vi "svfa_Process FRF (N pairs).vi"(0 "stimulus signals X [EUx]":waveform(dbl)[](array[waveform]), 1 "response signals Y [EUy]":waveform(dbl)[](array[waveform]), 2 "window":T9=1 items=["None"=0, "Hanning"=1, "Hamming"=2, "Blackman-Harris"=3, "Exact Blackman"=4, "Blackman"=5, "Flat Top"=6, "4 Term B-Harris "=7, "7 Term B-Harris"=8, "Low Sidelobe"=9, "Force - Exponential"=10, "Blackman Nuttall"=11, "Triangle"=30, "Bartlett-Hanning"=31, "Bohman"=32, "Parzen"=33, "Welch"=34, "Kaiser"=60, "Dolph-Chebyshev"=61, "Gaussian"=62], 3 "force/exp settings":T8={"force window [%]"=50.0, "exp window [%]"=10.0} {"exp window [%]" min=0.0 max=100.0 format="%.2f"; "force window [%]" min=0.0 max=100.0 format="%.2f"}, 4 "averaging parameters":T11={"averaging mode"=enum."No averaging", "weighting mode"=enum."Linear", "number of averages"=10, "linear mode"=enum."Auto restart"}, 5 "error in (no error)":errorcluster, 7 "processing control":T10(ring), 9 "FRF mode":enum16{"H1", "H2", "H3"}(ring), 11 "spectra info in":T1[](array[typedef]) {"x-axis units" items=["Time (s)"=0, "Frequency-CB (Hz)"=1, "Frequency-CPB (Hz)"=1248, "Frequency-Arbitrary (Hz)"=2357, "Quefrency (s)"=2, "Revolutions (rev)"=3, "Order"=4, "Speed (RPM)"=11, "Speed (rad/s)"=21, "Index"=65535]; "weighting filter" items=["Linear", "A-weighting", "B-weighting", "C-weighting", "ITU-R 468-4", "Dolby", "CCITT", "C-message", "Wb", "Wc", "Wd", "We", "Wf", "Wh", "Wj", "Wk", "Wm", "AES17 20 kHz lowpass", "AES17 40 kHz lowpass", "AES17 20 kHz highpass", "AES17 40 kHz highpass"]; "dB reference [EU]" format="%.2f"; "engineering units" items=["custom..."=0, "V"=1, "A"=21, "C"=30, "pC"=31, "s"=32, "-"=29, "Pa"=2, "N"=20, "g"=3, "m/s^2"=4, "m/s"=5, "m"=6, "mm/s"=12, "mm"=13, "micron/s"=14, "micron"=15, "in/s^2"=7, "in/s"=8, "in"=9, "mil/s"=10, "mil"=11, "rad/s^2"=16, "rad/s"=17, "rad"=18, "deg/s^2"=26, "deg/s"=27, "deg"=28, "RPM"=22, "cycle/s^2"=23, "Hz"=24, "cycle"=25, "strain"=19]; "spectral info"."window" items=["None "=0, "Hanning"=1, "Hamming"=2, "Blackman-Harris"=3, "Exact Blackman"=4, "Blackman"=5, "Flat Top"=6, "4 Term B-Harris "=7, "7 Term B-Harris"=8, "Low Sidelobe"=9, "Force - Exponential"=10, "Gaussian"=62]}) -> (8 "stimulus signals X [EUx] 2":waveform(dbl)[](array[waveform]), 10 "response signals Y [EUy] 2":waveform(dbl)[](array[waveform]), 12 "averages completed":dbl format="%.2f", 13 "processing control":T10(ring), 14 "complex responses [EUy/EUx]":T7(array[cluster]) {"complex spectrum" format="%.2f"; "df" format="%.2f"; "f0" format="%.2f"}, 16 "coherence":cluster{"f0":dbl, "df":dbl, "coherence":dbl[]}[](array[cluster]) {"coherence" format="%.2f"; "df" format="%.2f"; "f0" format="%.2f"}, 17 "averaging done":bool, 18 "spectra info out":T1[](array[typedef]) {"x-axis units" items=["Time (s)"=0, "Frequency-CB (Hz)"=1, "Frequency-CPB (Hz)"=1248, "Frequency-Arbitrary (Hz)"=2357, "Quefrency (s)"=2, "Revolutions (rev)"=3, "Order"=4, "Speed (RPM)"=11, "Speed (rad/s)"=21, "Index"=65535]; "weighting filter" items=["Linear", "A-weighting", "B-weighting", "C-weighting", "ITU-R 468-4", "Dolby", "CCITT", "C-message", "Wb", "Wc", "Wd", "We", "Wf", "Wh", "Wj", "Wk", "Wm", "AES17 20 kHz lowpass", "AES17 40 kHz lowpass", "AES17 20 kHz highpass", "AES17 40 kHz highpass"]; "dB reference [EU]" format="%.2f"; "engineering units" items=["custom..."=0, "V"=1, "A"=21, "C"=30, "pC"=31, "s"=32, "-"=29, "Pa"=2, "N"=20, "g"=3, "m/s^2"=4, "m/s"=5, "m"=6, "mm/s"=12, "mm"=13, "micron/s"=14, "micron"=15, "in/s^2"=7, "in/s"=8, "in"=9, "mil/s"=10, "mil"=11, "rad/s^2"=16, "rad/s"=17, "rad"=18, "deg/s^2"=26, "deg/s"=27, "deg"=28, "RPM"=22, "cycle/s^2"=23, "Hz"=24, "cycle"=25, "strain"=19]; "spectral info"."window" items=["None "=0, "Hanning"=1, "Hamming"=2, "Blackman-Harris"=3, "Exact Blackman"=4, "Blackman"=5, "Flat Top"=6, "4 Term B-Harris "=7, "7 Term B-Harris"=8, "Low Sidelobe"=9, "Force - Exponential"=10, "Gaussian"=62]}, 19 "error out":errorcluster)   [LabVIEW 2017]
uses:
  <vilib>/addons/_NISVFA/_Shared subVIs/Controls/svc_Window [Dual FFT].ctl
  <vilib>/addons/_NISVFA/_Shared subVIs/Controls/svc_Spectrum Info.ctl
  <vilib>/addons/_NISVFA/_Shared subVIs/Controls/svc_X-Axis Units.ctl
  <vilib>/addons/_NISVFA/_Shared subVIs/Controls/svc_Spectrum Type.ctl
  <vilib>/addons/_NISVFA/_Shared subVIs/Controls/svc_Engineering Units Text Ring.ctl
  <vilib>/addons/_NISVFA/_Shared subVIs/Controls/svc_Weighting Filter Text Ring.ctl
  <vilib>/addons/_NISVFA/_Shared subVIs/Controls/svc_Complimentary Spectrum Units.ctl
  <vilib>/addons/_NISVFA/_Shared subVIs/Windowing/svfa_Scaled Time Domain Window (N Ch).vi
  <vilib>/addons/_NISVFA/_Shared subVIs/Spectrum Averaging/svfa_Average Array (complex).vi
  <vilib>/addons/_NISVFA/_Shared subVIs/Spectrum Averaging/svfa_Average Array (real).vi
  <vilib>/addons/_NISVFA/_Shared subVIs/Windowing/svfa_Scaled Time Domain Window (1 Ch).vi
  <vilib>/addons/_NISVFA/_Shared subVIs/Windowing/svfa_Scaled Time Domain Window (Array).vi
  <vilib>/Analysis/4window.llb/Force Window.vi
  <vilib>/Analysis/4window.llb/Force Window (DBL).vi
  <vilib>/Analysis/4window.llb/Exponential Window.vi
  <vilib>/Analysis/4window.llb/Exponential Window (DBL).vi
  <vilib>/Utility/error.llb/Error Cluster From Error Code.vi
  <vilib>/Analysis/0measdsp.llb/Scaled Time Domain Window.vi
  <vilib>/Analysis/0measdsp.llb/Scaled Time Domain Window (DBL).vi
  <vilib>/addons/_NISVFA/_Spectrum Processing/subVIs/svfa_Spectrum Info Window to windowTd Type Def.vi
  <vilib>/addons/_NISVFA/_Shared subVIs/Common/svc_Window Parameters.vi
  <vilib>/addons/_NISVFA/_Shared subVIs/Common/svc_Get Window Info.vi
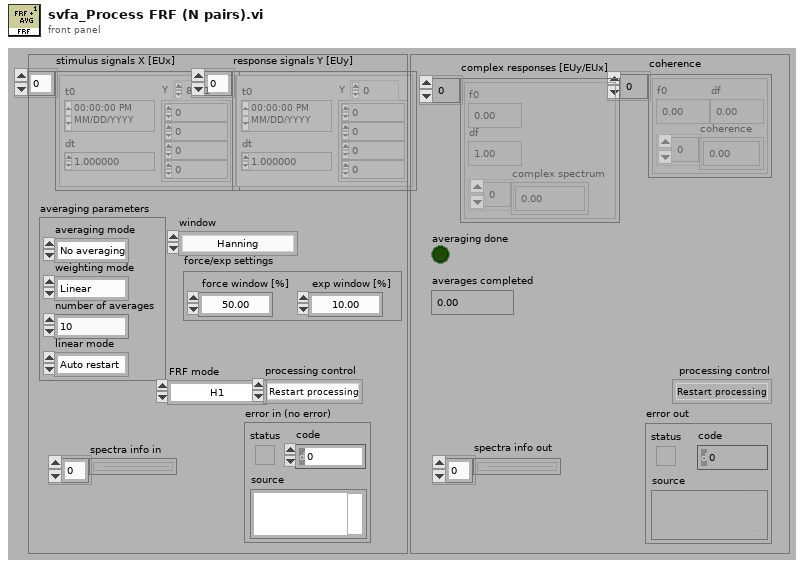
[diagram p1: front panel]
types:
  T1 = typedef "svc_Spectrum Info.ctl" = cluster{"channel name":string, "description":string, "x-axis units":T2, "spectral info":cluster{"spectrum type":T3, "linear/dB":enum16{"linear", "dB"}, "window":u16, "window size":i32, "FFT size":i32}, "engineering units":T4, "custom label":string, "dB reference [EU]":dbl, "peak units":enum16{"rms", "peak", "peak-peak"}, "weighting filter":T5, "spectral density?":bool, "unit label":string, "spectrum skewed?":bool, "complimentary spectrum units":T6}
  T2 = typedef "svc_X-Axis Units.ctl" = u16
  T3 = typedef "svc_Spectrum Type.ctl" = enum16{"FFT Spectrum [complex]", "Amplitude [Magnitude]", "Power [Magnitude^2]", "Cross Spectrum [complex]", "Frequency Response [Complex]"}
  T4 = typedef "svc_Engineering Units Text Ring.ctl" = u16
  T5 = typedef "svc_Weighting Filter Text Ring.ctl" = u16
  T6 = typedef "svc_Complimentary Spectrum Units.ctl" = enum16{"none", "radians", "degrees", "cycles", "imaginary"}
  T7 = cluster{"f0":dbl, "df":dbl, "complex spectrum":cdb[]}[]
  T8 = cluster{"force window [%]":dbl, "exp window [%]":dbl}
  T9 = typedef "svc_Window [Dual FFT].ctl" = u32
  T10 = enum16{"Restart processing", "Continue processing", "Skip processing"}
  T11 = cluster{"averaging mode":enum16{"No averaging", "Vector averaging", "RMS averaging", "Peak hold"}, "weighting mode":enum16{"Linear", "Exponential"}, "number of averages":u32, "linear mode":enum16{"One shot", "Auto restart"}}
  T12 = enum16{"No averaging", "Vector averaging", "RMS averaging", "Peak hold"}
  T13 = cluster{"f0":dbl, "df":dbl, "complex array":cdb[]}
  T14 = cluster{"f0":dbl, "df":dbl, "complex array":cdb[]}[]
  T15 = cluster{"complex spectrum":cluster{"f0":dbl, "df":dbl, "complex spectrum":cdb[]}, "spectrum info":T1}
  T16 = cluster{"f0":dbl, "df":dbl, "complex spectrum":cdb[]}
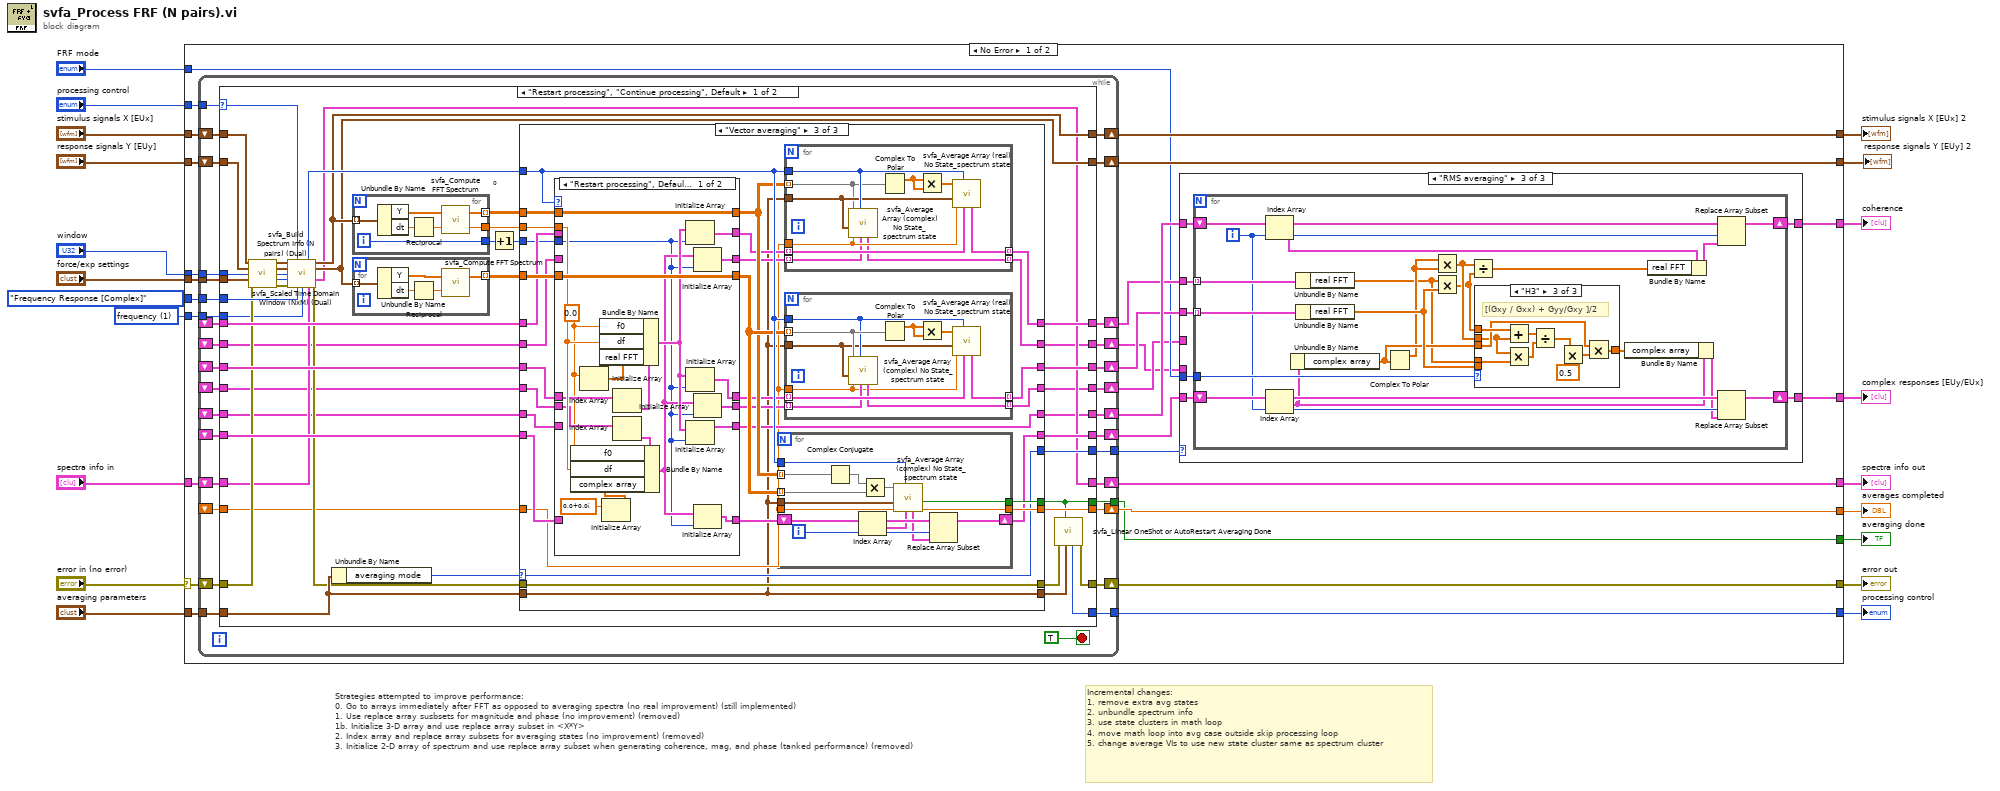
[diagram p0: block diagram]
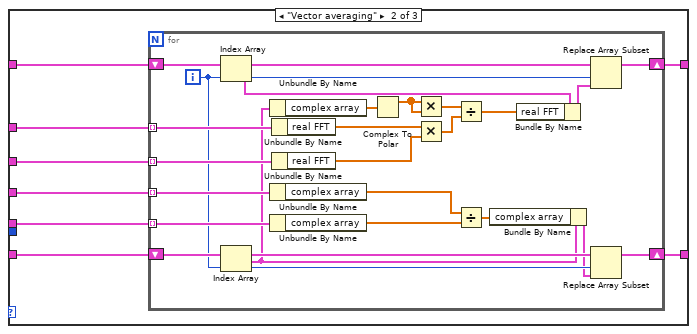
[diagram p3: hidden frame]
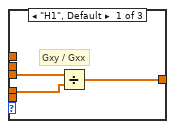
[diagram p4: hidden frame]
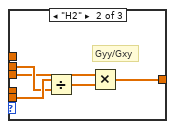
[diagram p5: hidden frame]
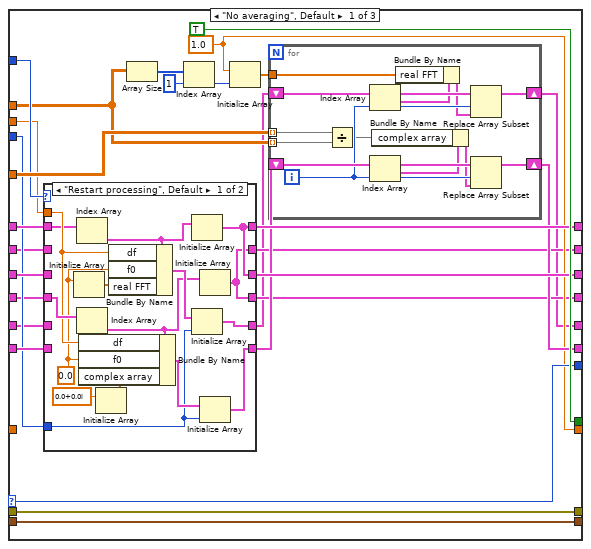
[diagram p6: hidden frame]
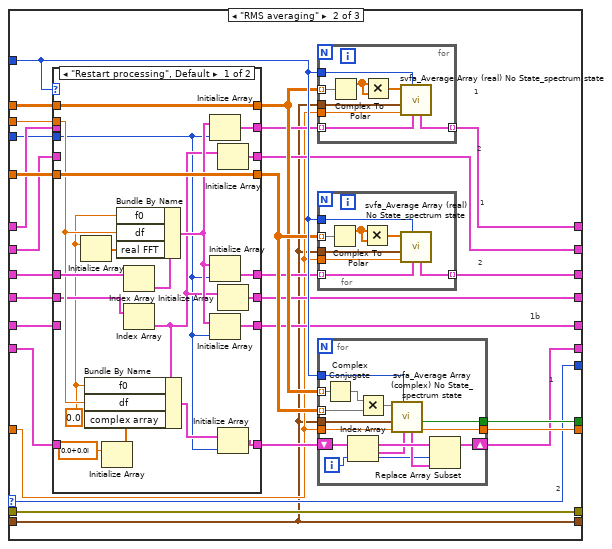
[diagram p8: hidden frame]
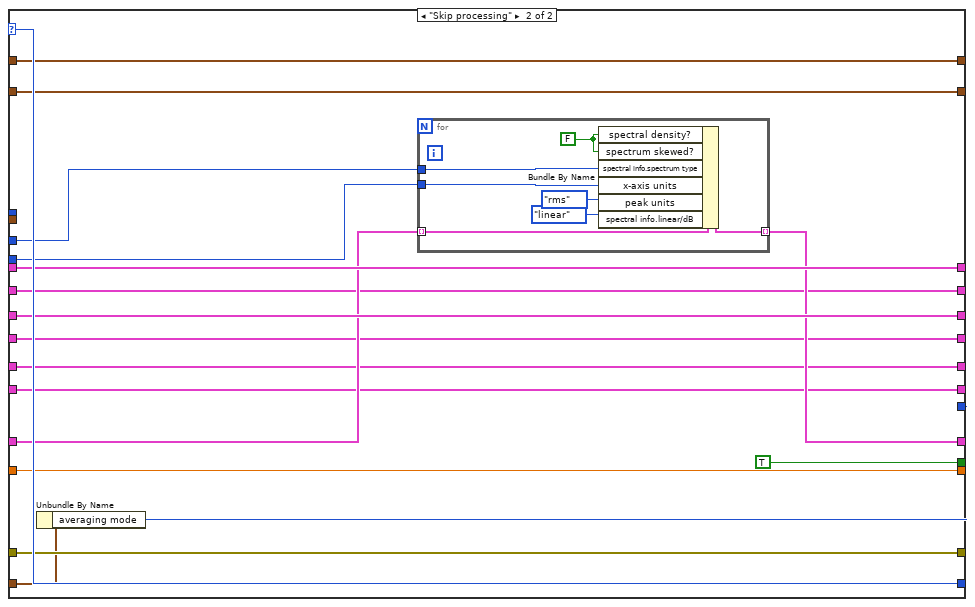
[diagram p11: hidden frame]
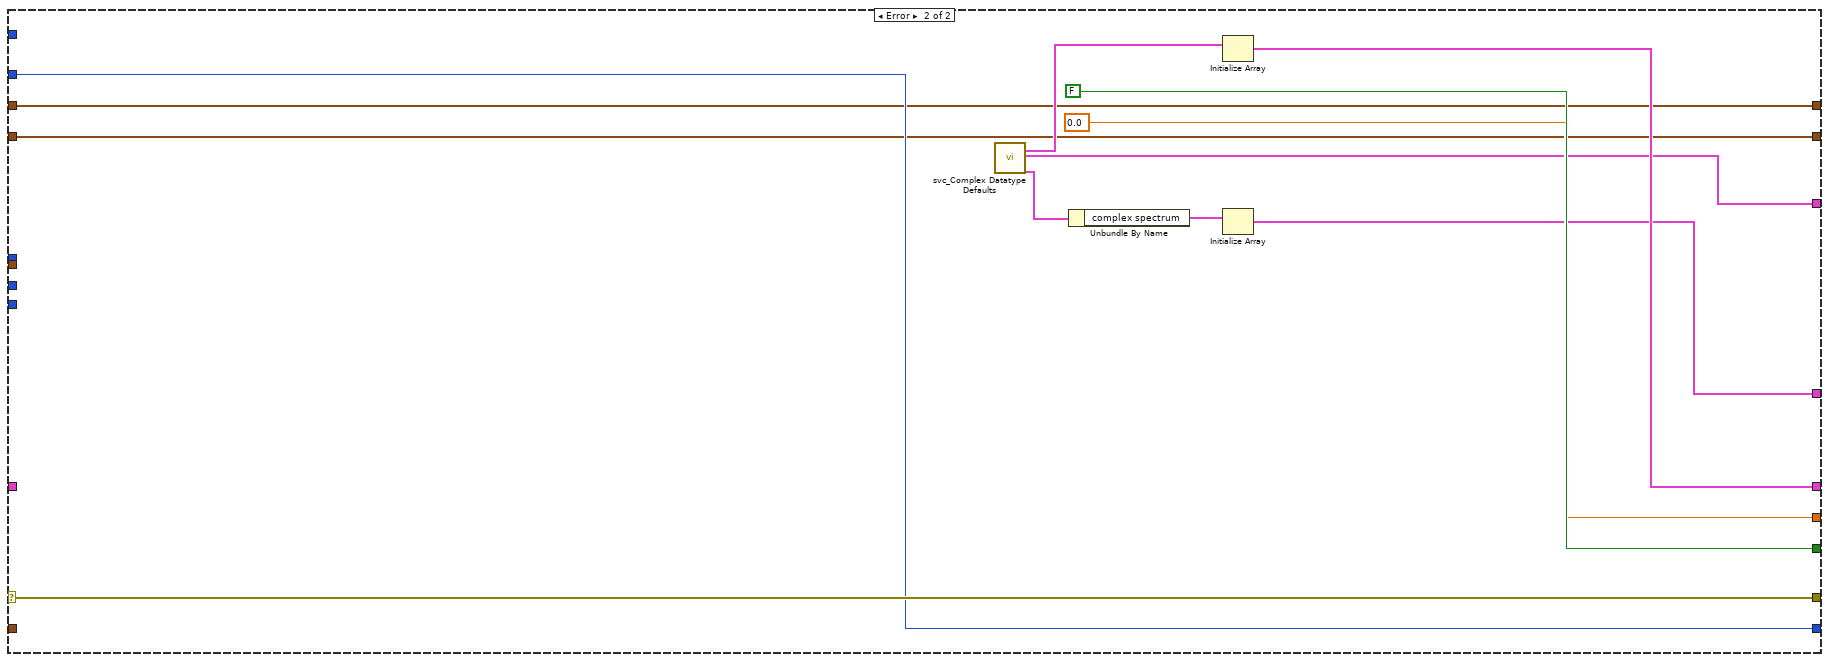
[diagram p12: hidden frame]
diagram:
  w6 = u16 1 items=["time"=0, "frequency"=1, "quefrency"=2, "revolutions"=3, "order"=4, "rpm"=11] ("x-axis units")
  # "Strategies attempted to improve performance:\n0. Go to arrays immediately after FFT as opposed to averaging spectra (no real improvement) (still implemented)\n1. Use replace array susbsets for magnitude and phase (no improvement) (removed)\n1b. Initialize 3-D array and use replace array subset in <X*Y>\n2. Index array and replace array subsets for averaging states (no improvement) (removed)\n3. Initialize 2-D array of spectrum and use replace array subset when generating coherence, mag, and phase (tanked performance) (removed)"
  # "Incremental changes:\n1. remove extra avg states\n2. unbundle spectrum info\n3. use state clusters in math loop\n4. move math loop into avg case outside skip processing loop\n5. change average VIs to use new state cluster same as spectrum cluster"
  n1 = case shown="No Error" "error in (no error)" {
    selector: "error in (no error)" -> [w44 w493]
    tunnel: [w38 w493] -> w20
    tunnel: "averaging parameters" -> [w47 _]
    tunnel: "stimulus signals X [EUx]" -> [w45 w484]
    tunnel: [w32 FALSE ("averaging done")] -> w16
    tunnel: [w46 0.0 ("averages completed")] -> w15
    tunnel: [w22 w485] -> w14
    tunnel: [w23 w482] -> w13
    tunnel: "FRF mode" -> [w26 _]
    tunnel: "processing control" -> [w43 w490]
    tunnel: [w39 w490] -> w10
    tunnel: "response signals Y [EUy]" -> [w42 w483]
    tunnel: "window" -> [w41 _]
    tunnel: "force/exp settings" -> [w40 _]
    tunnel: svc_Spectrum_Type."Frequency Response [Complex]" ("spectrum type") -> [w37 _]
    tunnel: w6 -> [w36 _]
    tunnel: [w35 w488] -> w5
    tunnel: [w34 w484] -> w4
    tunnel: [w33 w483] -> w3
    tunnel: "spectra info in" -> [w21 _]
    frame No Error {
      n2 = while {
        tunnel: [w149] -> w39
        tunnel: w40 -> [w150]
        tunnel: w41 -> [w151]
        tunnel: w43 -> [w146]
        tunnel: [w155] -> w32
        tunnel: w47 -> [w157]
        shift-right: [w145] -> w28
        shift-left: _ -> [w144]
        shift-right: [w127] -> w31
        shift-left: _ -> [w130]
        shift-right: [w143] -> w29
        shift-left: _ -> [w142]
        tunnel: w37 -> [w141]
        tunnel: w36 -> [w140]
        tunnel: [w137] -> w27
        shift-right: [w136] -> w34
        shift-left: w45 -> [w154]
        shift-right: [w135] -> w33
        shift-left: w42 -> [w152]
        shift-right: [w148] -> w38
        shift-left: w44 -> [w153]
        shift-right: [w138] -> w35
        shift-left: w21 -> [w139]
        shift-right: [w129] -> w24
        shift-left: _ -> [w132]
        shift-right: [w128] -> w25
        shift-left: _ -> [w131]
        shift-right: [w134] -> w30
        shift-left: _ -> [w133]
        shift-right: [w156] -> w46
        shift-left: _ -> [w126]
        stop <- TRUE stop-if-true
        n3 = case shown="\"Restart processing\", \"Continue processing\", Default" w146 {
          selector: w146 -> [w158 w474]
          tunnel: w157 -> [w190 w465]
          tunnel: [w202 w461] -> w156
          tunnel: [w201 TRUE ("averaging done")] -> w155
          tunnel: w153 -> [w176 w472]
          tunnel: w152 -> [w197 w462]
          tunnel: w151 -> [w196 _]
          tunnel: w150 -> [w186 _]
          tunnel: [w193 w474] -> w149
          tunnel: [w191 w472] -> w148
          tunnel: w154 -> [w198 w463]
          tunnel: [w185 w466] -> w134
          tunnel: [w184 w471] -> w145
          tunnel: w133 -> [w183 w466]
          tunnel: w144 -> [w182 w471]
          tunnel: [w181 w470] -> w143
          tunnel: w142 -> [w180 w470]
          tunnel: w141 -> [w179 w457]
          tunnel: w140 -> [w173 w467]
          tunnel: w139 -> [w172 w469]
          tunnel: [w166 w468] -> w138
          tunnel: [w171 w464] -> w137
          tunnel: [w168 w463] -> w136
          tunnel: [w167 w462] -> w135
          tunnel: w132 -> [w165 w460]
          tunnel: w131 -> [w164 w459]
          tunnel: w130 -> [w163 w458]
          tunnel: [w162 w460] -> w129
          tunnel: [w161 w459] -> w128
          tunnel: [w160 w458] -> w127
          tunnel: w126 -> [w159 w461]
          frame "Restart processing", "Continue processing", Default {
            # "0"
            n4 = call <vilib>:"svfa_Scaled Time Domain Window (NxM) (Dual).vi"("stimulus signals X [EUx]"=w198, "response signals Y [EUy]"=w197, "window"=w196, "Force - Exponential window settings"=w186, "error in (no error)"=w176) -> ("windowed stimulus signals X [EUx]"=w200:waveform(dbl)[], "windowed response signals Y [EUy]"=w199:waveform(dbl)[], "window"=w195:T9, "window size"=w188:i32, "error out"=w187:errorcluster)  [unwired: 6 in]
            n5 = call <vilib>:"svfa_Build Spectrum Info (N pairs) (Dual).vi"("stimulus signals X [EUx]"=w200, "processing control"=w158, "response signals Y [EUy]"=w199, "window"=w195, "window size"=w188, "error in (no error)"=w187, "spectrum type"=w179, "x-axis units"=w173, "spectra info in"=w172) -> ("dup processing control"=w192:T10, "dup stimulus signals X [EUx]"=w168:waveform(dbl)[], "response signals Y [EUy]"=w167:waveform(dbl)[], "spectra info out"=w166:T1[], "error out"=w169:errorcluster)  [unwired: 2 in]
            n6 = Unbundle By Name(w190) -> ("averaging mode"=w203:T12)
            n7 = for {
              tunnel: w168 -> [w215] mode=indexing
              tunnel: [w211] -> w189 mode=indexing
              tunnel: [w210] -> w170
              tunnel: [w209] -> w175
              i -> [w209]
              n8 = Unbundle By Name ("Get Waveform Components")(w215) -> ("Y"=w214:dbl[], "dt"=w213:dbl)
              n9 = Reciprocal(x=w213) -> (1/x=w212:dbl)
              n10 = call <vilib>:"svfa_Compute FFT Spectrum.vi"("sampling frequency [Hz]"=w212, "signal [EU]"=w214) -> ("df [Hz]"=w210:dbl, "FFT spectrum [EUrms]"=w211:cdb[])
            }
            n11 = for {
              tunnel: w167 -> [w208] mode=indexing
              tunnel: [w204] -> w178 mode=indexing
              n12 = Unbundle By Name ("Get Waveform Components")(w208) -> ("Y"=w207:dbl[], "dt"=w206:dbl)
              n13 = Reciprocal(x=w206) -> (1/x=w205:dbl)
              n14 = call <vilib>:"svfa_Compute FFT Spectrum.vi"("sampling frequency [Hz]"=w205, "signal [EU]"=w207) -> ("FFT spectrum [EUrms]"=w204:cdb[])  [unwired: 1 out]
            }
            n15 = Increment(x=w175) -> (x+1=w174:i32)
            n16 = case shown="\"Vector averaging\"" w203 {
              selector: w203 -> [w230 w289 w376]
              tunnel: [w241 w288 w375] -> w177
              tunnel: w169 -> [w241 w288 w375]
              tunnel: w190 -> [w242 w280 w365]
              tunnel: [TRUE ("averaging done") w306 w394] -> w201
              tunnel: w192 -> [w239 w304 w392]
              tunnel: [w225 w305 w393] -> w202
              tunnel: [w242 w280 w365] -> w194
              tunnel: w189 -> [w228 w302 w390]
              tunnel: w178 -> [w240 w303 w391]
              tunnel: [w231 w293 w377] -> w185
              tunnel: [w234 w291 w379] -> w184
              tunnel: w183 -> [w236 w296 w385]
              tunnel: w182 -> [w237 w295 w382]
              tunnel: [w235 w292 w380] -> w181
              tunnel: w180 -> [w238 w294 w383]
              tunnel: w170 -> [w229 w290 w378]
              tunnel: w174 -> [w233 w279 w381]
              tunnel: [w230 w289 w376] -> w171
              tunnel: w165 -> [w219 w286 w369]
              tunnel: w164 -> [w221 w284 w368]
              tunnel: w163 -> [w222 w282 w367]
              tunnel: [w220 w287 w373] -> w162
              tunnel: [w218 w285 w371] -> w161
              tunnel: [w216 w283 w370] -> w160
              tunnel: w159 -> [_ w281 w366]
              frame "No averaging", Default {
                w225 = 1.0 ("overwrite value")
                n17 = case shown="\"Restart processing\", Default" w239 {
                  tunnel: [w254 w265] -> w235
                  tunnel: w238 -> [w252 w265]
                  tunnel: [w254 w264] -> w234
                  tunnel: w237 -> [_ w264]
                  tunnel: [w259 w263] -> w232
                  tunnel: w236 -> [_ w263]
                  tunnel: w233 -> [w244 _]
                  tunnel: w229 -> [w257 _]
                  tunnel: w222 -> [_ w260]
                  tunnel: w221 -> [w258 w261]
                  tunnel: w219 -> [_ w262]
                  tunnel: [w253 w262] -> w220
                  tunnel: [w253 w261] -> w218
                  tunnel: [w255 w260] -> w217
                  frame "Restart processing", Default {
                    w250 = 0.0 ("f0")
                    n18 = Initialize Array(w250) -> (w251:dbl[])  [unwired: 1 in]
                    n19 = Index Array(array=w252) -> (element=w247:cluster{"f0":dbl, "df":dbl, "real FFT":dbl[]})  [unwired: 1 in]
                    n20 = Index Array(array=w258) -> (element=w246:T13)  [unwired: 1 in]
                    n21 = Initialize Array(cdb 0.0+0.0i ("element")) -> (w248:cdb[])  [unwired: 1 in]
                    n22 = Bundle By Name(cluster=w246, "df"=w257, "f0"=w250, "complex array"=w248) -> (w245:T13)
                    n23 = Bundle By Name(cluster=w247, "df"=w257, "f0"=w250, "real FFT"=w251) -> (w256:cluster{"f0":dbl, "df":dbl, "real FFT":dbl[]})
                    n24 = Initialize Array(w247) -> (w254:cluster{"f0":dbl, "df":dbl, "real FFT":dbl[]}[])  [unwired: 1 in]
                    n25 = Initialize Array(w256, w244) -> (w255:cluster{"f0":dbl, "df":dbl, "real FFT":dbl[]}[])
                    n26 = Initialize Array(w246) -> (w253:T14)  [unwired: 1 in]
                    n27 = Initialize Array(w245, w244) -> (w259:T14)
                  }
                  frame "Continue processing" {
                  }
                }
                n28 = Array Size(array=w228) -> (size(s)=w227:i32[])
                n29 = Index Array(array=w227, index=1) -> (element=w226:i32)
                n30 = Initialize Array(w225, w226) -> (w224:dbl[])
                n31 = for {
                  tunnel: w224 -> [w276]
                  tunnel: w228 -> [w278] mode=indexing
                  tunnel: w240 -> [w277] mode=indexing
                  shift-right: [w274] -> w231
                  shift-left: w232 -> [w275]
                  shift-right: [w271] -> w216
                  shift-left: w217 -> [w272]
                  i -> [w273]
                  n32 = Divide(x=w277, y=w278) -> (x/y=w270:cdb[])
                  n33 = Index Array(array=w272, index=w273) -> (element=w267:cluster{"f0":dbl, "df":dbl, "real FFT":dbl[]})
                  n34 = Index Array(array=w275, index=w273) -> (element=w268:T13)
                  n35 = Bundle By Name(cluster=w268, "complex array"=w270) -> (w269:T13)
                  n36 = Bundle By Name(cluster=w267, "real FFT"=w276) -> (w266:cluster{"f0":dbl, "df":dbl, "real FFT":dbl[]})
                  n37 = Replace Array Subset(array=w272, new element=w266, index=w273) -> (w271:cluster{"f0":dbl, "df":dbl, "real FFT":dbl[]}[])
                  n38 = Replace Array Subset(array=w275, new element=w269, index=w273) -> (w274:T14)
                }
              }
              frame "RMS averaging" {
                # "1"
                # "1b"
                # "2"
                # "2"
                # "2"
                # "1"
                # "1"
                n39 = case shown="\"Restart processing\", Default" w304 {
                  tunnel: w303 -> [w340 w345]
                  tunnel: w302 -> [w330 w348]
                  tunnel: [w340 w345] -> w301
                  tunnel: [w330 w348] -> w300
                  tunnel: [w339 w347] -> w299
                  tunnel: [w338 w346] -> w298
                  tunnel: [w337 w344] -> w297
                  tunnel: w296 -> [_ w347]
                  tunnel: w294 -> [_ w346]
                  tunnel: w295 -> [w336 w344]
                  tunnel: w279 -> [w321 _]
                  tunnel: w290 -> [w334 _]
                  tunnel: [w333 w343] -> w287
                  tunnel: w286 -> [_ w343]
                  tunnel: [w332 w342] -> w285
                  tunnel: w284 -> [w327 w342]
                  tunnel: [w331 w341] -> w283
                  tunnel: w282 -> [_ w341]
                  frame "Restart processing", Default {
                    w325 = 0.0 ("f0")
                    n40 = Initialize Array(w325) -> (w326:dbl[])  [unwired: 1 in]
                    n41 = Initialize Array(cdb 0.0+0.0i ("element")) -> (w323:cdb[])  [unwired: 1 in]
                    n42 = Index Array(array=w336) -> (element=w335:cluster{"f0":dbl, "df":dbl, "real FFT":dbl[]})  [unwired: 1 in]
                    n43 = Bundle By Name(cluster=w335, "f0"=w325, "df"=w334, "real FFT"=w326) -> (w329:cluster{"f0":dbl, "df":dbl, "real FFT":dbl[]})
                    n44 = Index Array(array=w327) -> (element=w322:T13)  [unwired: 1 in]
                    n45 = Bundle By Name(cluster=w322, "f0"=w325, "df"=w334, "complex array"=w323) -> (w328:T13)
                    n46 = Initialize Array(w329, w321) -> (w338:cluster{"f0":dbl, "df":dbl, "real FFT":dbl[]}[])
                    n47 = Initialize Array(w329, w321) -> (w337:cluster{"f0":dbl, "df":dbl, "real FFT":dbl[]}[])
                    n48 = Initialize Array(w329, w321) -> (w331:cluster{"f0":dbl, "df":dbl, "real FFT":dbl[]}[])
                    n49 = Initialize Array(w322) -> (w333:T14)  [unwired: 1 in]
                    n50 = Initialize Array(w322) -> (w332:T14)  [unwired: 1 in]
                    n51 = Initialize Array(w328, w321) -> (w339:T14)
                  }
                  frame "Continue processing", "Skip processing" {
                  }
                }
                n52 = for {
                  tunnel: w300 -> [w361] mode=indexing
                  tunnel: w304 -> [w364]
                  tunnel: w281 -> [w359]
                  tunnel: w298 -> [w357] mode=indexing
                  tunnel: [w358] -> w292 mode=indexing
                  tunnel: w280 -> [w360]
                  n53 = Complex To Polar(r * e^(i*theta)=w361) -> (r=w363:dbl[])  [unwired: 1 out]
                  n54 = Multiply(x=w363, y=w363) -> (x*y=w362:dbl[])
                  n55 = call <vilib>:"svfa_Average Array (real) No State_spectrum state.vi"("previous avg real spectrum"=w357, "processing control"=w364, "averages completed"=w359, "averaging parameters"=w360, "array"=w362) -> ("new avg real spectrum"=w358:cluster{"f0":dbl, "df":dbl, "real FFT":dbl[]})  [unwired: 4 in, 2 out]
                }
                n56 = for {
                  tunnel: w301 -> [w353] mode=indexing
                  tunnel: w304 -> [w356]
                  tunnel: w280 -> [w355]
                  tunnel: w297 -> [w351] mode=indexing
                  tunnel: [w350] -> w291 mode=indexing
                  tunnel: w281 -> [w349]
                  n57 = Complex To Polar(r * e^(i*theta)=w353) -> (r=w354:dbl[])  [unwired: 1 out]
                  n58 = Multiply(x=w354, y=w354) -> (x*y=w352:dbl[])
                  n59 = call <vilib>:"svfa_Average Array (real) No State_spectrum state.vi"("previous avg real spectrum"=w351, "processing control"=w356, "averages completed"=w349, "averaging parameters"=w355, "array"=w352) -> ("new avg real spectrum"=w350:cluster{"f0":dbl, "df":dbl, "real FFT":dbl[]})  [unwired: 4 in, 2 out]
                }
                n60 = for {
                  tunnel: w304 -> [w318]
                  tunnel: w280 -> [w320]
                  tunnel: w301 -> [w315] mode=indexing
                  tunnel: [w317] -> w306
                  tunnel: [w316] -> w305
                  shift-right: [w313] -> w293
                  shift-left: w299 -> [w314]
                  tunnel: w281 -> [w310]
                  tunnel: w300 -> [w308] mode=indexing
                  i -> [w307]
                  n61 = Complex Conjugate(1:w308) -> (0:w309:cdb[])
                  n62 = Index Array(array=w314, index=w307) -> (element=w311:T13)
                  n63 = Multiply(x=w309, y=w315) -> (x*y=w319:cdb[])
                  n64 = call <vilib>:"svfa_Average Array (complex) No State_spectrum state.vi"("previous avg complex spectrum"=w311, "processing control"=w318, "averages completed in"=w310, "averaging parameters"=w320, "array"=w319) -> ("averages completed out"=w316:dbl, "averaging done"=w317:bool, "avg complex spectrum"=w312:T13)  [unwired: 4 in]
                  n65 = Replace Array Subset(array=w314, new element=w312, index=w307) -> (w313:T14)
                }
              }
              frame "Vector averaging" {
                n66 = case shown="\"Restart processing\", Default" w392 {
                  tunnel: w391 -> [w414 w422]
                  tunnel: w390 -> [w404 w421]
                  tunnel: [w414 w422] -> w389
                  tunnel: [w404 w421] -> w388
                  tunnel: [w413 w420] -> w387
                  tunnel: [w412 w419] -> w386
                  tunnel: w385 -> [_ w420]
                  tunnel: w383 -> [_ w419]
                  tunnel: [w411 w418] -> w384
                  tunnel: w382 -> [w401 w418]
                  tunnel: w381 -> [w395 _]
                  tunnel: w378 -> [w406 _]
                  tunnel: [w409 w417] -> w374
                  tunnel: [w408 w416] -> w372
                  tunnel: [w407 w415] -> w370
                  tunnel: w369 -> [_ w417]
                  tunnel: w368 -> [w400 w416]
                  tunnel: w367 -> [_ w415]
                  frame "Restart processing", Default {
                    w399 = 0.0 ("f0")
                    n67 = Initialize Array(w399) -> (w398:dbl[])  [unwired: 1 in]
                    n68 = Initialize Array(cdb 0.0+0.0i ("element")) -> (w396:cdb[])  [unwired: 1 in]
                    n69 = Index Array(array=w401) -> (element=w410:cluster{"f0":dbl, "df":dbl, "real FFT":dbl[]})  [unwired: 1 in]
                    n70 = Bundle By Name(cluster=w410, "f0"=w399, "df"=w406, "real FFT"=w398) -> (w403:cluster{"f0":dbl, "df":dbl, "real FFT":dbl[]})
                    n71 = Index Array(array=w400) -> (element=w405:T13)  [unwired: 1 in]
                    n72 = Bundle By Name(cluster=w405, "f0"=w399, "df"=w406, "complex array"=w396) -> (w402:T13)
                    n73 = Initialize Array(w403, w395) -> (w412:cluster{"f0":dbl, "df":dbl, "real FFT":dbl[]}[])
                    n74 = Initialize Array(w403, w395) -> (w411:cluster{"f0":dbl, "df":dbl, "real FFT":dbl[]}[])
                    n75 = Initialize Array(w403, w395) -> (w407:cluster{"f0":dbl, "df":dbl, "real FFT":dbl[]}[])
                    n76 = Initialize Array(w402, w395) -> (w409:T14)
                    n77 = Initialize Array(w402, w395) -> (w408:T14)
                    n78 = Initialize Array(w402, w395) -> (w413:T14)
                  }
                  frame "Continue processing", "Skip processing" {
                  }
                }
                n79 = for {
                  tunnel: w388 -> [w436] mode=indexing
                  tunnel: w389 -> [w435] mode=indexing
                  tunnel: w392 -> [w434]
                  tunnel: w365 -> [w433]
                  tunnel: [w432] -> w394
                  tunnel: [w431] -> w393
                  shift-right: [w429] -> w377
                  shift-left: w387 -> [w430]
                  tunnel: w366 -> [w427]
                  i -> [w428]
                  n80 = Complex Conjugate(1:w436) -> (0:w426:cdb[])
                  n81 = Index Array(array=w430, index=w428) -> (element=w423:T13)
                  n82 = Multiply(x=w426, y=w435) -> (x*y=w425:cdb[])
                  n83 = call <vilib>:"svfa_Average Array (complex) No State_spectrum state.vi"("previous avg complex spectrum"=w423, "processing control"=w434, "averages completed in"=w427, "averaging parameters"=w433, "array"=w425) -> ("averages completed out"=w431:dbl, "averaging done"=w432:bool, "avg complex spectrum"=w424:T13)  [unwired: 4 in]
                  n84 = Replace Array Subset(array=w430, new element=w424, index=w428) -> (w429:T14)
                }
                n85 = for {
                  tunnel: w388 -> [w447] mode=indexing
                  tunnel: w392 -> [w456]
                  tunnel: w386 -> [w452] mode=indexing
                  tunnel: [w451] -> w380 mode=indexing
                  tunnel: w374 -> [w449] mode=indexing
                  tunnel: [w448] -> w373 mode=indexing
                  tunnel: w366 -> [w453]
                  tunnel: w365 -> [w450]
                  n86 = call <vilib>:"svfa_Average Array (complex) No State_spectrum state.vi"("previous avg complex spectrum"=w449, "processing control"=w456, "averages completed in"=w453, "averaging parameters"=w450, "array"=w447) -> ("avg complex spectrum"=w448:T13)  [unwired: 4 in, 2 out]
                  n87 = Complex To Polar(r * e^(i*theta)=w447) -> (r=w455:dbl[])  [unwired: 1 out]
                  n88 = Multiply(x=w455, y=w455) -> (x*y=w454:dbl[])
                  n89 = call <vilib>:"svfa_Average Array (real) No State_spectrum state.vi"("previous avg real spectrum"=w452, "processing control"=w456, "averages completed"=w453, "averaging parameters"=w450, "array"=w454) -> ("new avg real spectrum"=w451:cluster{"f0":dbl, "df":dbl, "real FFT":dbl[]})  [unwired: 4 in, 2 out]
                }
                n90 = for {
                  tunnel: w389 -> [w446] mode=indexing
                  tunnel: w392 -> [w444]
                  tunnel: w365 -> [w437]
                  tunnel: [w445] -> w379 mode=indexing
                  tunnel: w384 -> [w441] mode=indexing
                  tunnel: w372 -> [w440] mode=indexing
                  tunnel: [w439] -> w371 mode=indexing
                  tunnel: w366 -> [w438]
                  n91 = call <vilib>:"svfa_Average Array (complex) No State_spectrum state.vi"("previous avg complex spectrum"=w440, "processing control"=w444, "averages completed in"=w438, "averaging parameters"=w437, "array"=w446) -> ("avg complex spectrum"=w439:T13)  [unwired: 4 in, 2 out]
                  n92 = Complex To Polar(r * e^(i*theta)=w446) -> (r=w443:dbl[])  [unwired: 1 out]
                  n93 = Multiply(x=w443, y=w443) -> (x*y=w442:dbl[])
                  n94 = call <vilib>:"svfa_Average Array (real) No State_spectrum state.vi"("previous avg real spectrum"=w441, "processing control"=w444, "averages completed"=w438, "averaging parameters"=w437, "array"=w442) -> ("new avg real spectrum"=w445:cluster{"f0":dbl, "df":dbl, "real FFT":dbl[]})  [unwired: 4 in, 2 out]
                }
              }
            }
            n95 = call <vilib>:"svfa_Linear OneShot or AutoRestart Averaging Done.vi"("averaging parameters"=w194, "averaging done"=w201, "error in (no error)"=w177) -> ("error out"=w191:errorcluster, "processing control"=w193:T10)  [unwired: 7 in]
          }
          frame "Skip processing" {
            n96 = Unbundle By Name(w465) -> ("averaging mode"=w464:T12)
            n97 = for {
              tunnel: w469 -> [w478] mode=indexing
              tunnel: [w477] -> w468 mode=indexing
              tunnel: w467 -> [w476]
              tunnel: w457 -> [w475]
              w480 = FALSE ("spectral density?")
              n98 = Bundle By Name(cluster=w478, "spectral density?"=w480, "spectrum skewed?"=w480, "spectral info.spectrum type"=w475, "x-axis units"=w476, "peak units"=enum16{"rms", "peak", "peak-peak"}."rms", "spectral info.linear/dB"=enum16{"linear", "dB"}."linear") -> (w477:T1)
            }
          }
        }
      }
      n99 = case shown="\"RMS averaging\"" w27 {
        tunnel: w30 -> [w48 w57 w85]
        tunnel: w28 -> [_ w56 w86]
        tunnel: w29 -> [_ w55 w87]
        tunnel: [w49 w51 w83] -> w23
        tunnel: [w48 w50 w84] -> w22
        tunnel: w26 -> [_ _ w82]
        tunnel: w31 -> [w49 w52 w81]
        tunnel: w24 -> [_ w54 _]
        tunnel: w25 -> [_ w53 _]
        frame "No averaging", Default {
        }
        frame "Vector averaging" {
          n100 = for {
            tunnel: w55 -> [w80] mode=indexing
            tunnel: w56 -> [w79] mode=indexing
            tunnel: w53 -> [w77] mode=indexing
            tunnel: w54 -> [w76] mode=indexing
            shift-right: [w73] -> w51
            shift-left: w52 -> [w75]
            shift-right: [w72] -> w50
            shift-left: w57 -> [w78]
            i -> [w74]
            n101 = Index Array(array=w75, index=w74) -> (element=w66:cluster{"f0":dbl, "df":dbl, "real FFT":dbl[]})
            n102 = Index Array(array=w78, index=w74) -> (element=w62:T13)
            n103 = Unbundle By Name(w62) -> ("complex array"=w68:cdb[])
            n104 = Unbundle By Name(w77) -> ("complex array"=w67:cdb[])
            n105 = Unbundle By Name(w76) -> ("complex array"=w58:cdb[])
            n106 = Unbundle By Name(w80) -> ("real FFT"=w59:dbl[])
            n107 = Unbundle By Name(w79) -> ("real FFT"=w69:dbl[])
            n108 = Complex To Polar(r * e^(i*theta)=w68) -> (r=w60:dbl[])  [unwired: 1 out]
            n109 = Multiply(x=w60, y=w60) -> (x*y=w71:dbl[])
            n110 = Multiply(x=w59, y=w69) -> (x*y=w70:dbl[])
            n111 = Divide(x=w71, y=w70) -> (x/y=w64:dbl[])
            n112 = Divide(x=w67, y=w58) -> (x/y=w61:cdb[])
            n113 = Bundle By Name(cluster=w62, "complex array"=w61) -> (w63:T13)
            n114 = Bundle By Name(cluster=w66, "real FFT"=w64) -> (w65:cluster{"f0":dbl, "df":dbl, "real FFT":dbl[]})
            n115 = Replace Array Subset(array=w75, new element=w65, index=w74) -> (w73:cluster{"f0":dbl, "df":dbl, "real FFT":dbl[]}[])
            n116 = Replace Array Subset(array=w78, new element=w63, index=w74) -> (w72:T14)
          }
        }
        frame "RMS averaging" {
          n117 = for {
            tunnel: w87 -> [w104] mode=indexing
            tunnel: w86 -> [w103] mode=indexing
            tunnel: w82 -> [w102]
            shift-right: [w107] -> w83
            shift-left: w81 -> [w101]
            shift-right: [w106] -> w84
            shift-left: w85 -> [w105]
            i -> [w100]
            n118 = Index Array(array=w101, index=w100) -> (element=w98:cluster{"f0":dbl, "df":dbl, "real FFT":dbl[]})
            n119 = Index Array(array=w105, index=w100) -> (element=w94:T13)
            n120 = Unbundle By Name(w94) -> ("complex array"=w93:cdb[])
            n121 = Unbundle By Name(w104) -> ("real FFT"=w89:dbl[])
            n122 = Unbundle By Name(w103) -> ("real FFT"=w99:dbl[])
            n123 = Complex To Polar(r * e^(i*theta)=w93) -> (r=w90:dbl[])  [unwired: 1 out]
            n124 = Multiply(x=w90, y=w90) -> (x*y=w91:dbl[])
            n125 = Multiply(x=w89, y=w99) -> (x*y=w88:dbl[])
            n126 = Divide(x=w91, y=w88) -> (x/y=w97:dbl[])
            n127 = case shown="\"H3\"" w102 {
              tunnel: [w110 w111 w123] -> w92
              tunnel: w89 -> [w109 _ w119]
              tunnel: w99 -> [_ w115 _]
              tunnel: w93 -> [w108 w112 w117]
              tunnel: w91 -> [_ w114 w116]
              tunnel: w88 -> [_ _ w122]
              frame "H1", Default {
                # "Gxy / Gxx"
                n128 = Divide(x=w108, y=w109) -> (x/y=w110:cdb[])
              }
              frame "H2" {
                # "Gyy/Gxy"
                n129 = Divide(x=w115, y=w114) -> (x/y=w113:dbl[])
                n130 = Multiply(x=w112, y=w113) -> (x*y=w111:cdb[])
              }
              frame "H3" {
                # "[(Gxy / Gxx) + Gyy/Gxy ]/2"
                n131 = Add(x=w122, y=w116) -> (x+y=w121:dbl[])
                n132 = Multiply(x=w116, y=w119) -> (x*y=w118:dbl[])
                n133 = Divide(x=w121, y=w118) -> (x/y=w120:dbl[])
                n134 = Multiply(x=w120, y=0.5) -> (x*y=w124:dbl[])
                n135 = Multiply(x=w117, y=w124) -> (x*y=w123:cdb[])
              }
            }
            n136 = Bundle By Name(cluster=w94, "complex array"=w92) -> (w95:T13)
            n137 = Bundle By Name(cluster=w98, "real FFT"=w97) -> (w96:cluster{"f0":dbl, "df":dbl, "real FFT":dbl[]})
            n138 = Replace Array Subset(array=w101, new element=w96, index=w100) -> (w107:cluster{"f0":dbl, "df":dbl, "real FFT":dbl[]}[])
            n139 = Replace Array Subset(array=w105, new element=w95, index=w100) -> (w106:T14)
          }
        }
      }
    }
    frame Error {
      n140 = call <vilib>:"svc_Complex Datatype Defaults.vi"() -> ("dead spectrum info"=w489:T1, "empty array of spectra"=w482:cluster{"f0":dbl, "df":dbl, "magnitude":dbl[]}[], "complex spectrum"=w487:T15)  [unwired: 11 in, 6 out]
      n141 = Unbundle By Name(w487) -> ("complex spectrum"=w486:T16)
      n142 = Initialize Array(w489) -> (w488:T1[])  [unwired: 1 in]
      n143 = Initialize Array(w486) -> (w485:T7)  [unwired: 1 in]
    }
  }
  "error out" <- w20
  "averages completed" <- w15
  "averaging done" <- w16
  "complex responses [EUy/EUx]" <- w14
  "coherence" <- w13
  "processing control" <- w10
  "spectra info out" <- w5
  "stimulus signals X [EUx] 2" <- w4
  "response signals Y [EUy] 2" <- w3
